vi "Change Image Directory.vi"(8 "error in":errorcluster, 10 "Image Dir":path, 11 "TSC Button Editor in":refnum<class "TSC Button Editor.lvclass">) -> (0 "error out":errorcluster, 3 "TSC Button Editor out":refnum<class "TSC Button Editor.lvclass">, 4 "Images":T1(array[cluster]))   [LabVIEW 2021, in "TSC Button Editor.lvclass"]
doc: "This VI will change the image directory and load the images from that location.\n\n<b>Code Developed By:</b> +\nDaniel Coons +\nTechnology Service Corporation +\nwww.tsc.com/atcs"
uses:
  TSC Button Editor.lvclass
  TSC Button Editor.lvclass/TSC Button Editor.ctl
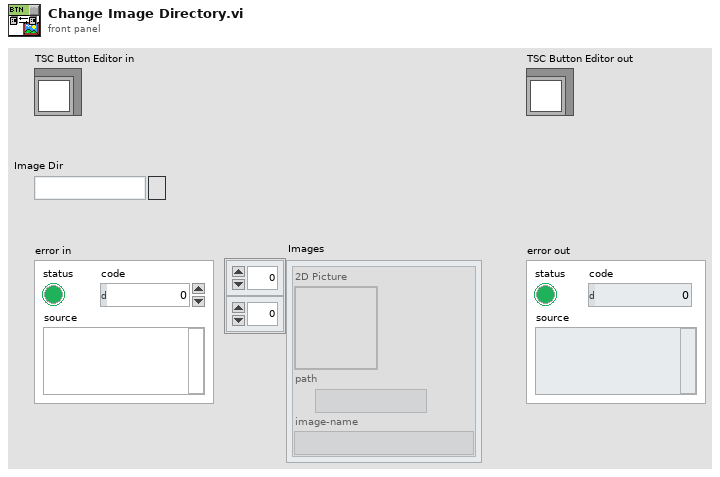
[diagram p1: front panel]
types:
  T1 = cluster{"2D Picture":picture, "path":path, "image-name":string}[][]
  T2 = enum16{"open", "replace", "create", "open or create", "replace or create", "replace or create with confirmation"}
  T3 = cluster{"2D Picture":picture, "path":path, "image-name":string}[]
  T4 = cluster{"2D Picture":picture, "path":path, "image-name":string}
  T5 = typedef "imagedata.ctl" = cluster{"image type":i32, "image depth":i32, "image":u8[], "mask":u8[], "colors":u32[], "Rectangle":cluster{"left":i16, "top":i16, "right":i16, "bottom":i16}}
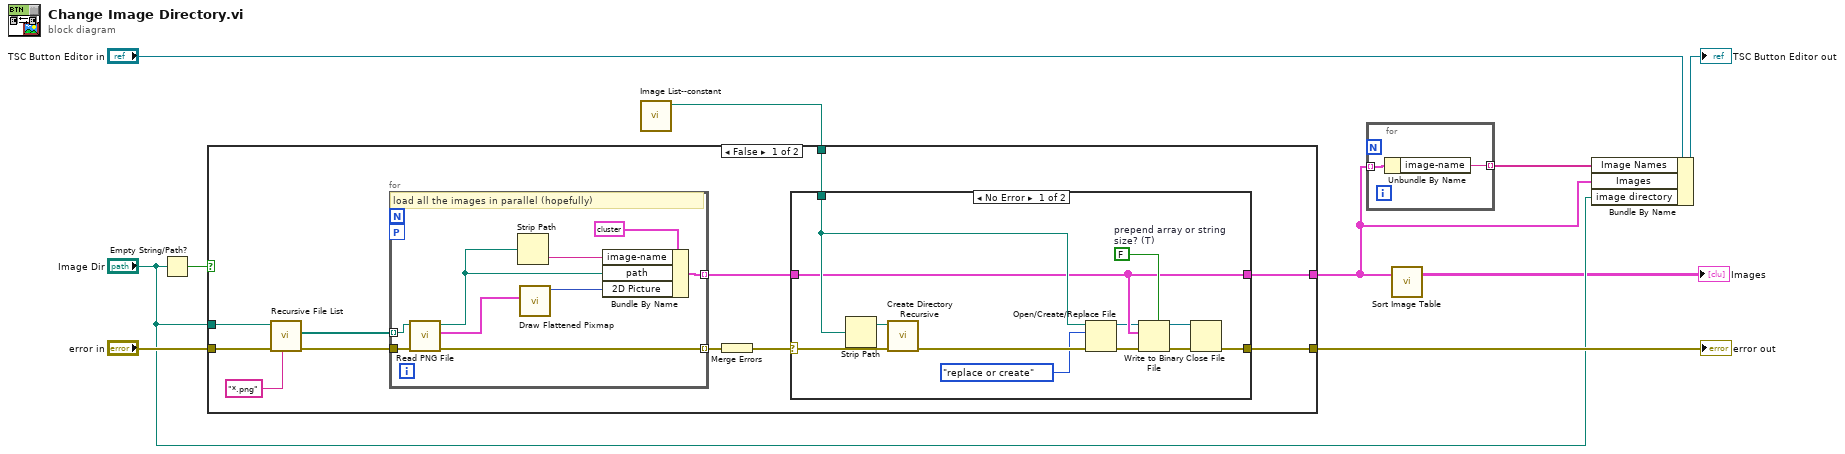
[diagram p0: block diagram]
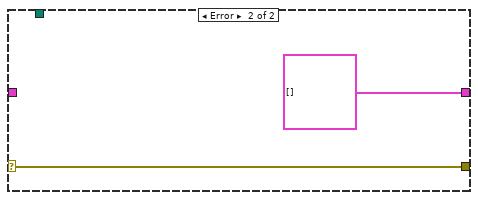
[diagram p2: hidden frame]
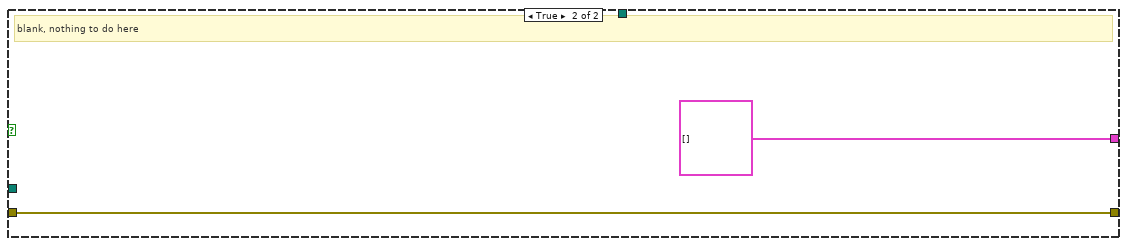
[diagram p3: hidden frame]
diagram:
  n1 = Empty String/Path?(string/path="Image Dir") -> (empty?=w5:bool)
  n2 = call "Image List--constant.vi"() -> ("image-list"=w4:path)  [unwired: 11 in]
  n3 = case shown="False" w5 {
    tunnel: "error in" -> [w21 w46]
    tunnel: [w19 w46] -> w9
    tunnel: "Image Dir" -> [w16 _]
    tunnel: [w12 T3 []] -> w1
    tunnel: w4 -> [w11 _]
    frame False {
      n4 = call <vilib>:"Recursive File List.vi"("pattern"="*.png", "error in (no error)"=w21, "Folder Path"=w16) -> ("error out"=w20:errorcluster, "All Files in Dir"=w15:path[])  [unwired: 4 in, 3 out]
      n5 = for {
        tunnel: w15 -> [w42] mode=indexing
        tunnel: [w40] -> w13 mode=indexing
        workers-P: _ -> [_]
        tunnel: w20 -> [w44]
        tunnel: [w43] -> w14 mode=indexing
        # "load all the images in parallel (hopefully)"
        n6 = call <vilib>:"Read PNG File.vi"("error in (no error)"=w44, "path to PNG file"=w42) -> ("error out"=w43:errorcluster, "image data"=w41:T5, "path"=w37:path)  [unwired: 7 in]
        n7 = Strip Path(path=w37) -> (name=w36:string)  [unwired: 1 out]
        n8 = call <vilib>:"Draw Flattened Pixmap.vi"("image data"=w41) -> ("new picture"=w38:picture)  [unwired: 8 in]
        n9 = Bundle By Name(cluster=T4 {"2D Picture"=bytes[0], "path"=path "", "image-name"=""} ("Cluster"), "image-name"=w36, "path"=w37, "2D Picture"=w38) -> (w40:T4)
      }
      n10 = Merge Errors(w14) -> (w18:errorcluster)
      n11 = case shown="No Error" w18 {
        selector: w18 -> [w32 w35]
        tunnel: [w29 w35] -> w19
        tunnel: w13 -> [w24 _]
        tunnel: [w24 T3 []] -> w12
        tunnel: w11 -> [w26 _]
        frame No Error {
          w25 = FALSE  # prepend array or string size? (T)
          n12 = Strip Path(path=w26) -> (stripped path=w27:path)  [unwired: 1 out]
          n13 = call <vilib>:"Create Directory Recursive.vi"("error in (no error)"=w32, "directory"=w27) -> ("error out"=w31:errorcluster)  [unwired: 3 in, 2 out]
          n14 = Open/Create/Replace File(file path (use dialog)=w26, error in=w31, operation (0:open)=T2."replace or create") -> (refnum out=w23:refnum<file>, error out=w33:errorcluster)  [unwired: 3 in, 1 out]
          n15 = Write to Binary File(file (use dialog)=w23, data=w24, error in=w33, 5:w25) -> (refnum out=w22:refnum<file>, error out=w30:errorcluster)  [unwired: 2 in, 1 out]
          n16 = Close File(refnum=w22, error in=w30) -> (error out=w29:errorcluster)  [unwired: 1 out]
        }
        frame Error {
        }
      }
    }
    frame True {
      # "blank, nothing to do here"
    }
  }
  "error out" <- w9
  n17 = for {
    tunnel: w1 -> [w48] mode=indexing
    tunnel: [w47] -> w6 mode=indexing
    n18 = Unbundle By Name(w48) -> ("image-name"=w47:string)
  }
  n19 = call "Sort Image Table.vi"("Images in"=w1) -> ("Images out"=→"Images":T1)  [unwired: 2 in]
  n20 = Bundle By Name(cluster="TSC Button Editor in", "Image Names"=w6, "Images"=w1, "image directory"="Image Dir") -> (→"TSC Button Editor out":refnum<class "TSC Button Editor.lvclass">)
